vi "Get Active UUTs.vi"(8 "error in (no error)":errorcluster, 11 "Application in":refnum<class "Application.lvclass">) -> (0 "error out":errorcluster, 2 "Active Positions":u32[](array[numeric]), 3 "Application out":refnum<class "Application.lvclass">)   [LabVIEW 2017, in "Application.lvlib" / "Application.lvclass"]
doc: "Returns the positions of all UUTs in a \"Ready\" state."
uses:
  Application.lvclass
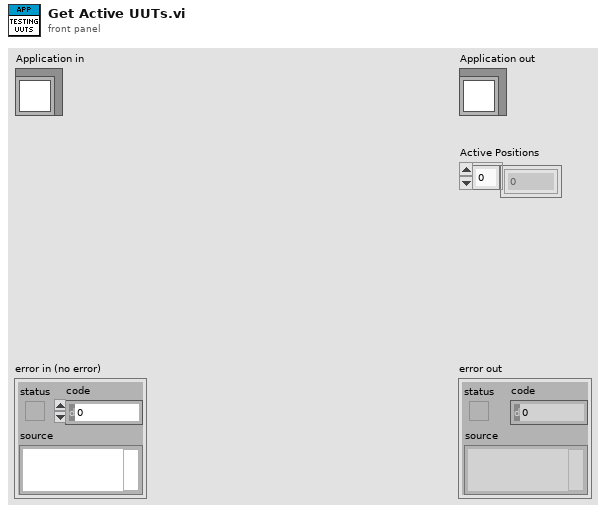
[diagram p1: front panel]
types:
  T1 = cluster{"Serial Number Reference":refnum<vi>, "Status Message Reference":refnum<vi>, "Position":u32}[]
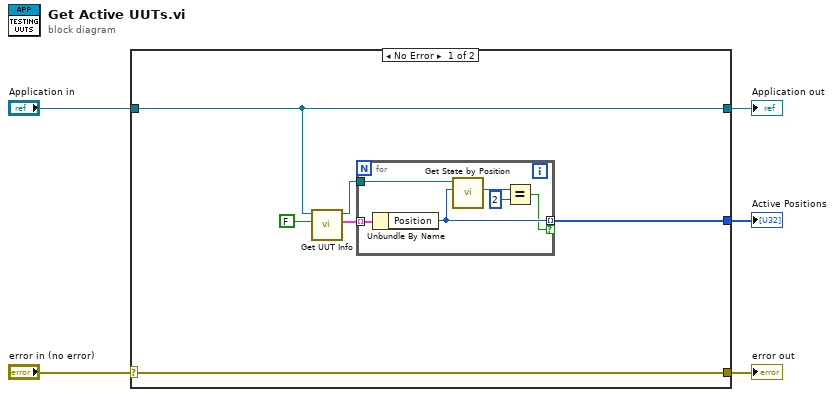
[diagram p0: block diagram]
diagram:
  n1 = case shown="No Error" "error in (no error)" {
    selector: "error in (no error)" -> [w11 w19]
    tunnel: [w11 w19] -> w4
    tunnel: [w9 w18] -> w2
    tunnel: "Application in" -> [w9 w18]
    tunnel: [w10 _] -> w1
    frame No Error {
      n2 = call-dynamic "Get UUT Info.vi"("Scanned Only (false)"=FALSE, "Application in"=w9) -> ("All UUTs"=w7:T1, "Application out"=w8:refnum<class "Application.lvclass">)  [unwired: 7 in, 1 out]
      n3 = for {
        tunnel: w7 -> [w17] mode=indexing
        tunnel: w8 -> [w16]
        tunnel: [w15] -> w10 mode=indexing if=w14
        n4 = Unbundle By Name(w17) -> ("Position"=w15:u32)
        n5 = call-dynamic "Get State by Position.vi"("Position"=w15, "Application in"=w16) -> ("State"=w13:u32)  [unwired: 7 in, 2 out]
        n6 = Equal?(x=w13, y=u32 2) -> (x = y?=w14:bool)
      }
    }
    frame Error {
    }
  }
  "error out" <- w4
  "Application out" <- w2
  "Active Positions" <- w1
